vi "Wykres.vi"(9 "index":i32, 11 "Y":dbl) -> (3 "output array":dbl[](array[numeric]))   [LabVIEW 2020]
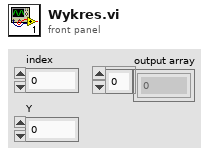
[diagram p1: front panel]
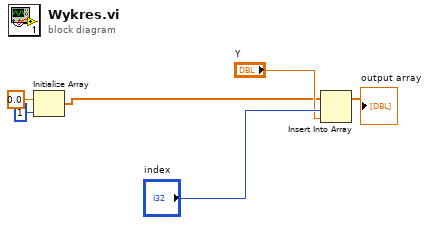
[diagram p0: block diagram]
diagram:
  n1 = Initialize Array(0.0 ("element"), 1 ("dimension size")) -> (w1:dbl[])
  n2 = Insert Into Array(array=w1, index="index", new element="Y") -> (→"output array":dbl[])
